vi "run.vi"(8 "error in (no error)":errorcluster, 11 "DL090215DataCollection in":refnum<class "DataCollectionDL090215.lvclass">=refnum) -> (0 "error out":errorcluster, 3 "DL090215DataCollection out":refnum<class "DataCollectionDL090215.lvclass">)   [LabVIEW 2010, in "DataCollectionDL090215.lvclass"]
uses:
  DataCollectionDL090215.lvclass
  GenericDataCollection/GenericDataCollection/GenericDataCollection.lvclass
  common/classes/ErrorController/ErrorController/ErrorController.lvclass
  DataCollectionDL091104Scaffold/DataCollectionDL091104Scaffold/DataCollectionDL091104Scaffold.lvclass
  common/classes/GenericComponent/GenericComponent/GenericComponent.lvclass
  common/xcontrols/XSettings/XSettings/XSettings.xctl
  main/labview_source/controls/undock_button.ctl
panel:
  in  "enforce settings?":bool
  in  "button:undock":T1
  in  "Tab Control":enum32{"User", "Debug", "About"}(tab)
  in  "Which channels to save?":bool[](array[boolean])
  in  "write header?":bool=TRUE
  in  "autosave?":bool=TRUE
  in  "frame":i32(slide)=1 min=1 step=1 scale=1.0..1.1
  in  "play button":bool
  in  "fps":dbl=5.0
  in  "notebook import string ref":refnum<k21>
  in  "OME header import string ref":refnum<k21>
  in  "XSettings":refnum<class "GenericComponent.lvclass">(xcontrol)
  out "finished?":bool=TRUE
  out "event loop counter":i32
  # "Shared Variable Engine binding paths"
  # "DataCollectionDL090215"
  # "Implemented by: \nDominik Langer, University of Zurich"
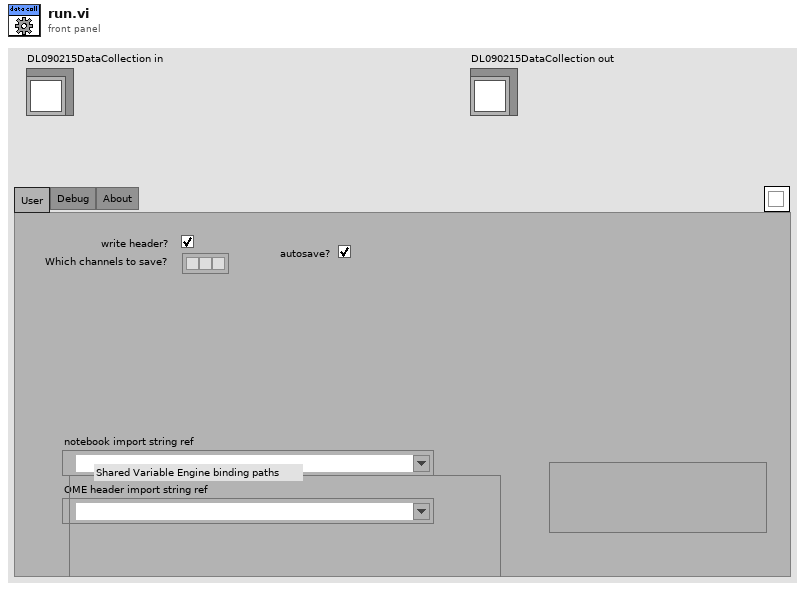
[diagram p1: front panel]
types:
  T1 = typedef "undock_button.ctl" = bool
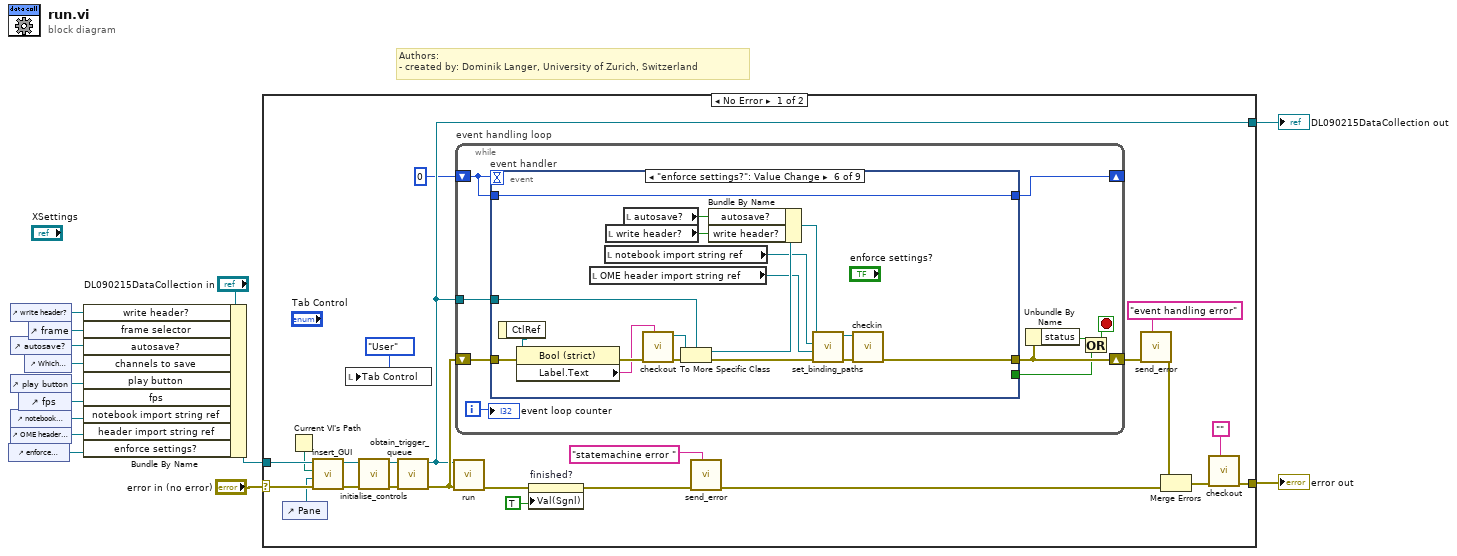
[diagram p0: block diagram]
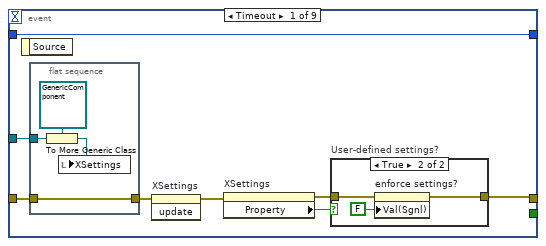
[diagram p2: hidden frame]
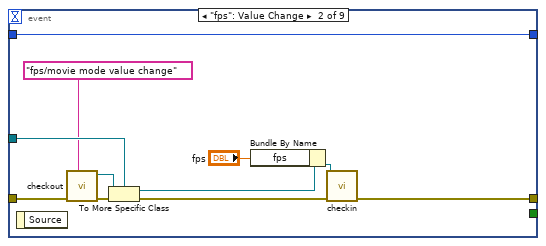
[diagram p4: hidden frame]
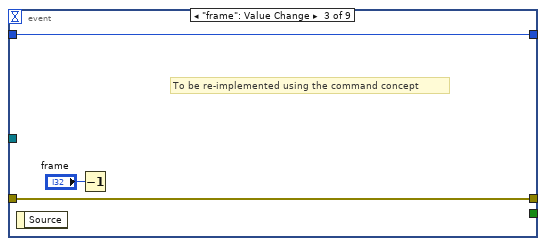
[diagram p5: hidden frame]
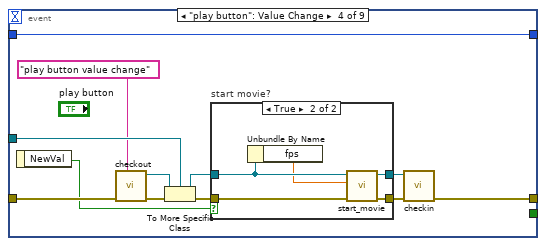
[diagram p6: hidden frame]
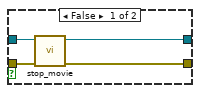
[diagram p7: hidden frame]
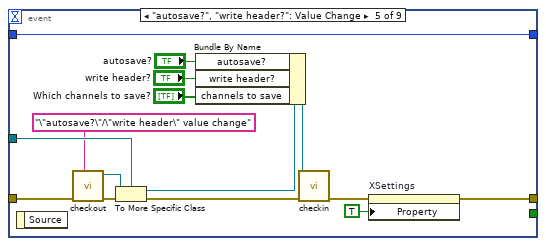
[diagram p8: hidden frame]
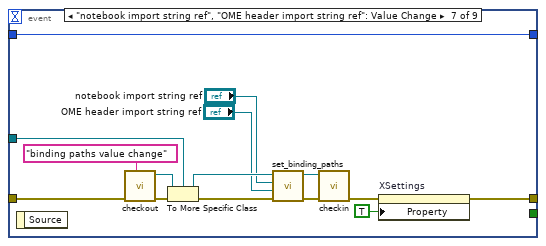
[diagram p9: hidden frame]
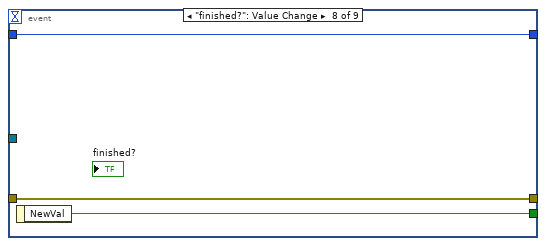
[diagram p10: hidden frame]
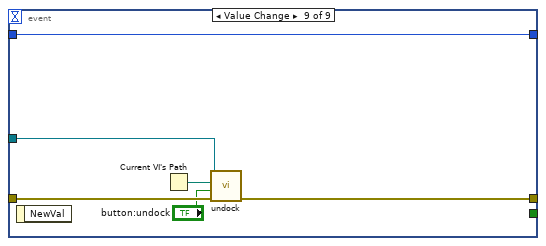
[diagram p11: hidden frame]
diagram:
  # "Authors: \n- created by: Dominik Langer, University of Zurich, Switzerland"
  n1 = control-ref of="enforce settings?"() -> (w1:refnum<vi>)
  n2 = control-ref of="write header?"() -> (w5:refnum<vi>)
  n3 = control-ref of="autosave?"() -> (w8:refnum<vi>)
  n4 = control-ref of="play button"() -> (w7:refnum<vi>)
  n5 = control-ref of="notebook import string ref"() -> (w4:refnum<vi>)
  n6 = control-ref of="OME header import string ref"() -> (w3:refnum<vi>)
  n7 = control-ref of="fps"() -> (w6:refnum<vi>)
  n8 = control-ref of="Which channels to save?"() -> (w2:refnum<vi>)
  n9 = control-ref of="frame"() -> (w9:refnum<vi>)
  n10 = Bundle By Name(cluster="DL090215DataCollection in", "write header?"=w5, "frame selector"=w9, "autosave?"=w8, "channels to save"=w2, "play button"=w7, "fps"=w6, "notebook import string ref"=w4, "header import string ref"=w3, "enforce settings?"=w1) -> (w10:refnum<class "DataCollectionDL090215.lvclass">)
  n11 = case shown="No Error" "error in (no error)" {
    selector: "error in (no error)" -> [w31 w156]
    tunnel: [w20 w156] -> w13
    tunnel: [w32 w155] -> w12
    tunnel: w10 -> [w30 w155]
    frame No Error {
      n12 = control-ref of="Pane"() -> (w25:refnum<vi>)
      n13 = Current VI's Path() -> (path=w29:path)
      n14 = call-dynamic "insert_GUI.vi"("error in (no error)"=w31, "Pane"=w25, "VI path"=w29, "GenericComponent in"=w30) -> ("error out"=w28:errorcluster, "GenericComponent out"=w27:refnum<class "DataCollectionDL090215.lvclass">)  [unwired: 6 in]
      n15 = local write "Tab Control"(enum32{"User", "Debug", "About"}."User" ("Tab Control")) -> ()
      n16 = call-dynamic "initialise_controls.vi"("error in (no error)"=w28, "DL090215DataCollection in"=w27) -> ("error out"=w23:errorcluster, "DL090215DataCollection out"=w24:refnum<class "DataCollectionDL090215.lvclass">)  [unwired: 8 in]
      n17 = call-dynamic "obtain_trigger_queue.vi"("error in (no error)"=w23, "GenericPlugin in"=w24) -> ("error out"=w33:errorcluster, "GenericPlugin out"=w32:refnum<class "DataCollectionDL090215.lvclass">)  [unwired: 7 in, 1 out]
      n18 = call-parent "run.vi"("error in (no error)"=w33, "DataCollectionDL091104Scaffold.lvclass out"=w32) -> ("error out"=w35:errorcluster)  [unwired: 8 in, 1 out]
      n19 = while "event handling loop" {
        tunnel: w32 -> [w45]
        shift-right: [w43] -> w22
        shift-left: w33 -> [w46]
        shift-right: [w38] -> _
        shift-left: 0 -> [w39]
        i -> [w44]
        stop <- w40 stop-if-true
        n20 = event "event handler" shown="[5] \"enforce settings?\": Value Change" {
          selector: _ -> [_ _ _ _ _ _ _ _ _]
          dyn-events: _ -> [_ _ _ _ _ _ _ _ _]
          timeout: w39 -> [_ _ _ _ _ _ _ _ _]
          tunnel: w46 -> [w53 w72 w75 w88 w112 w128 w140 w148 w154]
          tunnel: [w47 w66 w75 w87 w100 w119 w131 w148 w153] -> w43
          tunnel: [_ _ _ _ _ _ _ w147 _] -> w42
          tunnel: w45 -> [w54 w71 _ w86 w111 w124 w138 _ w152]
          tunnel: w39 -> [w52 w63 w74 w77 w102 w130 w134 w146 w149]
          tunnel: [w52 w63 w74 w77 w102 w130 w134 w146 w149] -> w38
          event Timeout {
            n21 = event-data() -> ()  [unwired: 2 out]
            n22 = flat-sequence {
              tunnel: w54 -> [w61]
              tunnel: w53 -> [w59]
              tunnel: [w59] -> w51
              frame #0 {
                n23 = To More Generic Class(target class=refnum<class "GenericComponent.lvclass"> refnum ("GenericComponent.lvclass"), reference=w61) -> (generic class reference=w60:refnum<class "GenericComponent.lvclass">)
                n24 = local write "XSettings"(w60) -> ()
              }
            }
            n25 = invoke on="XSettings" class="XSettings (strict)" method="update"(error in=w51) -> (error out=w50:errorcluster)  [unwired: 2 in, 2 out]
            n26 = property on="XSettings" class="XSettings (strict)"(error in=w50) -> (error out=w49:errorcluster, "Property"=w48:bool)  [unwired: 1 in, 1 out]
            n27 = case "User-defined settings?" shown="True" w48 {
              tunnel: w49 -> [w55 w57]
              tunnel: [w55 w56] -> w47
              frame False {
              }
              frame True {
                n28 = property on="enforce settings?" class="Bool (strict)"(error in=w57, "Val(Sgnl)"=FALSE ("Value (Signaling)")) -> (error out=w56:errorcluster)  [unwired: 1 in, 1 out]
              }
            }
          }
          event "fps": Value Change {
            n29 = event-data() -> ()  [unwired: 2 out]
            n30 = call "checkout.vi"("locked by?"="fps/movie mode value change", "error in (no error)"=w72) -> ("error out"=w73:errorcluster, "GenericDataCollection out"=w70:refnum<class "GenericDataCollection.lvclass">)  [unwired: 8 out]
            n31 = To More Specific Class(target class=w71, reference=w70, error in=w73) -> (specific class reference=w69:refnum<class "DataCollectionDL090215.lvclass">, error out=w67:errorcluster)
            n32 = Bundle By Name(cluster=w69, "fps"="fps") -> (w65:refnum<class "DataCollectionDL090215.lvclass">)
            n33 = call-dynamic "checkin.vi"("error in (no error)"=w67, "GenericDataCollection in"=w65) -> ("error out"=w66:errorcluster)  [unwired: 8 in, 1 out]
          }
          event "frame": Value Change {
            # "To be re-implemented using the command concept"
            n34 = event-data() -> ()  [unwired: 2 out]
            n35 = Decrement(x="frame") -> ()  [unwired: 1 out]
          }
          event "play button": Value Change {
            n36 = event-data() -> ("NewVal"=w79:bool)  [unwired: 1 out]
            n37 = call "checkout.vi"("locked by?"="play button value change", "error in (no error)"=w88) -> ("error out"=w85:errorcluster, "GenericDataCollection out"=w84:refnum<class "GenericDataCollection.lvclass">)  [unwired: 8 out]
            n38 = To More Specific Class(target class=w86, reference=w84, error in=w85) -> (specific class reference=w80:refnum<class "DataCollectionDL090215.lvclass">, error out=w83:errorcluster)
            n39 = case "start movie?" shown="True" w79 {
              tunnel: w83 -> [w92 w97]
              tunnel: [w91 w96] -> w82
              tunnel: [w90 w95] -> w81
              tunnel: w80 -> [w89 w94]
              frame False {
                n40 = call-dynamic "stop_movie.vi"("error in (no error)"=w92, "DataCollectionDL091104Scaffold in"=w89) -> ("error out"=w91:errorcluster, "DataCollectionDL091104Scaffold out"=w90:refnum<class "DataCollectionDL090215.lvclass">)  [unwired: 8 in]
              }
              frame True {
                n41 = Unbundle By Name(w94) -> ("fps"=w93:dbl)
                n42 = call-dynamic "start_movie.vi"("error in (no error)"=w97, "frames per second"=w93, "DataCollectionDL091104Scaffold in"=w94) -> ("error out"=w96:errorcluster, "DataCollectionDL091104Scaffold out"=w95:refnum<class "DataCollectionDL090215.lvclass">)  [unwired: 7 in]
              }
            }
            n43 = call-dynamic "checkin.vi"("error in (no error)"=w82, "GenericDataCollection in"=w81) -> ("error out"=w87:errorcluster)  [unwired: 8 in, 1 out]
          }
          event "autosave?", "write header?": Value Change {
            n44 = event-data() -> ()  [unwired: 2 out]
            n45 = call "checkout.vi"("locked by?"="\"autosave?\"/\"write header\" value change", "error in (no error)"=w112) -> ("error out"=w110:errorcluster, "GenericDataCollection out"=w109:refnum<class "GenericDataCollection.lvclass">)  [unwired: 8 out]
            n46 = To More Specific Class(target class=w111, reference=w109, error in=w110) -> (specific class reference=w107:refnum<class "DataCollectionDL090215.lvclass">, error out=w108:errorcluster)
            n47 = Bundle By Name(cluster=w107, "autosave?"="autosave?", "write header?"="write header?", "channels to save"="Which channels to save?") -> (w106:refnum<class "DataCollectionDL090215.lvclass">)
            n48 = call-dynamic "checkin.vi"("error in (no error)"=w108, "GenericDataCollection in"=w106) -> ("error out"=w101:errorcluster)  [unwired: 8 in, 1 out]
            n49 = property on="XSettings" class="XSettings (strict)"(error in=w101, "Property"=TRUE ("is user-defined?")) -> (error out=w100:errorcluster)  [unwired: 1 in, 1 out]
          }
          event "enforce settings?": Value Change {
            n50 = event-data() -> ("CtlRef"=w129:refnum<vi>)  [unwired: 1 out]
            n51 = property class="Bool (strict)"(reference=w129, error in=w128) -> (error out=w127:errorcluster, "Label.Text"=w126:string)  [unwired: 1 out]
            n52 = local read "OME header import string ref"() -> (w113:refnum<k21>)
            n53 = local read "notebook import string ref"() -> (w114:refnum<k21>)
            n54 = local read "write header?"() -> (w121:bool)
            n55 = local read "autosave?"() -> (w120:bool)
            n56 = call "checkout.vi"("locked by?"=w126, "error in (no error)"=w127) -> ("error out"=w123:errorcluster, "GenericDataCollection out"=w125:refnum<class "GenericDataCollection.lvclass">)  [unwired: 8 in]
            n57 = To More Specific Class(target class=w124, reference=w125, error in=w123) -> (specific class reference=w122:refnum<class "DataCollectionDL090215.lvclass">, error out=w116:errorcluster)
            n58 = Bundle By Name(cluster=w122, "autosave?"=w120, "write header?"=w121) -> (w118:refnum<class "DataCollectionDL090215.lvclass">)
            n59 = call-dynamic "set_binding_paths.vi"("error in (no error)"=w116, "OME header import string ref"=w113, "notebook import string ref"=w114, "DataCollectionDL090215 in"=w118) -> ("error out"=w115:errorcluster, "DataCollectionDL090215 out"=w117:refnum<class "DataCollectionDL090215.lvclass">)  [unwired: 6 in]
            n60 = call-dynamic "checkin.vi"("error in (no error)"=w115, "GenericDataCollection in"=w117) -> ("error out"=w119:errorcluster)  [unwired: 8 in, 1 out]
          }
          event "notebook import string ref", "OME header import string ref": Value Change {
            n61 = event-data() -> ()  [unwired: 2 out]
            n62 = call "checkout.vi"("locked by?"="binding paths value change", "error in (no error)"=w140) -> ("error out"=w145:errorcluster, "GenericDataCollection out"=w144:refnum<class "GenericDataCollection.lvclass">)  [unwired: 8 out]
            n63 = To More Specific Class(target class=w138, reference=w144, error in=w145) -> (specific class reference=w139:refnum<class "DataCollectionDL090215.lvclass">, error out=w142:errorcluster)
            n64 = call-dynamic "set_binding_paths.vi"("error in (no error)"=w142, "OME header import string ref"="OME header import string ref", "notebook import string ref"="notebook import string ref", "DataCollectionDL090215 in"=w139) -> ("error out"=w141:errorcluster, "DataCollectionDL090215 out"=w137:refnum<class "DataCollectionDL090215.lvclass">)  [unwired: 6 in]
            n65 = call-dynamic "checkin.vi"("error in (no error)"=w141, "GenericDataCollection in"=w137) -> ("error out"=w132:errorcluster)  [unwired: 8 in, 1 out]
            n66 = property on="XSettings" class="XSettings (strict)"(error in=w132, "Property"=TRUE ("is user-defined?")) -> (error out=w131:errorcluster)  [unwired: 1 in, 1 out]
          }
          event "finished?": Value Change {
            n67 = event-data() -> ("NewVal"=w147:bool)  [unwired: 1 out]
          }
          event Value Change {
            n68 = event-data() -> ()  [unwired: 2 out]
            n69 = Current VI's Path() -> (path=w150:path)
            n70 = call-dynamic "undock.vi"("error in (no error)"=w154, "undock?"="button:undock", "VI path"=w150, "component in"=w152) -> ("error out"=w153:errorcluster)  [unwired: 6 in, 1 out]
          }
        }
        n71 = Unbundle By Name(w43) -> ("status"=w41:bool)
        n72 = Or(x=w41, y=w42) -> (x .or. y?=w40:bool)
        "event loop counter" <- w44
      }
      n73 = property on="finished?" class="Bool (strict)"(error in=w35, "Val(Sgnl)"=TRUE) -> (error out=w19:errorcluster)  [unwired: 1 in, 1 out]
      n74 = call "send_error.vi"("additional message"="statemachine error ", "error in (no error)"=w19) -> ("error out"=w18:errorcluster)  [unwired: 9 in]
      n75 = call "send_error.vi"("additional message"="event handling error", "error in (no error)"=w22) -> ("error out"=w21:errorcluster)  [unwired: 9 in]
      n76 = Merge Errors(w21, w18) -> (w37:errorcluster)
      n77 = call "checkout.vi"("locked by?"="", "error in (no error)"=w37) -> ("error out"=w20:errorcluster)  [unwired: 9 out]
    }
    frame Error {
    }
  }
  "error out" <- w13
  "DL090215DataCollection out" <- w12
